vi "Read Offset.vi"(8 "error in (no error)":errorcluster, 11 "Parameter in":refnum<class "Parameter.lvclass">) -> (0 "error out":errorcluster, 2 "Offset":dbl, 3 "Parameter out":refnum<class "Parameter.lvclass">)   [LabVIEW 2013, in "Parameter.lvclass"]
uses:
  Parameter.lvclass
  Parameter.lvclass/Parameter.ctl
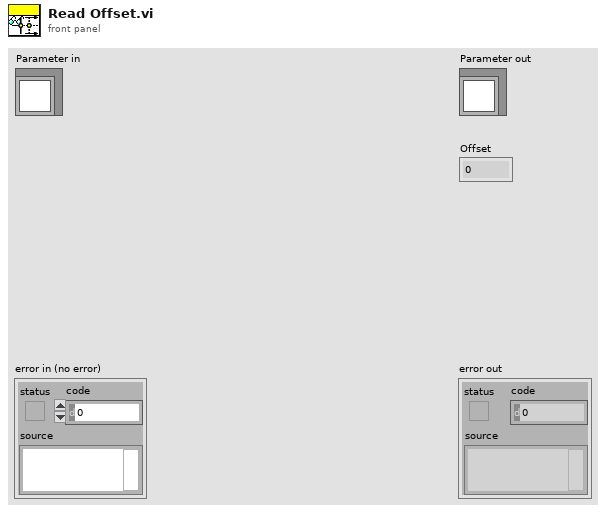
[diagram p1: front panel]
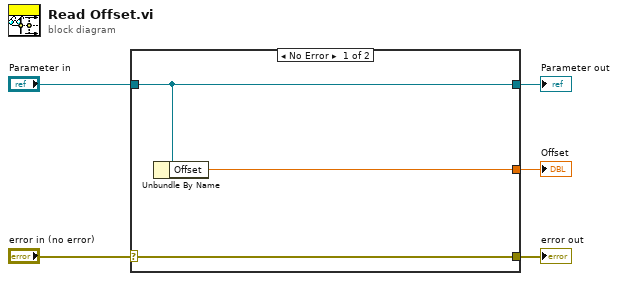
[diagram p0: block diagram]
diagram:
  n1 = case shown="No Error" "error in (no error)" {
    selector: "error in (no error)" -> [w8 w9]
    tunnel: [w8 w9] -> w4
    tunnel: [w7 w10] -> w2
    tunnel: "Parameter in" -> [w7 w10]
    tunnel: [w6 _] -> w1
    frame No Error {
      n2 = Unbundle By Name(w7) -> ("Offset"=w6:dbl)
    }
    frame Error {
    }
  }
  "error out" <- w4
  "Parameter out" <- w2
  "Offset" <- w1
